vi "Instrument.TestLauncher.vi"(8 "error in (no error)":errorcluster, 10 "Debug Mode?":bool=TRUE) -> (0 "error out":errorcluster)   [LabVIEW 2019, in "Instrument.lvclass"]
uses:
  Instrument.lvclass
  <vilib>/JKI/JKI SMO/SMO/Typedefs/SMOState --Enum.ctl
  C:/Program Files (x86)/National Instruments/LabVIEW 2019/vi.lib/JKI/JKI SMO/SMO/SMO.lvclass
  <vilib>/JKI/JKI SMO/SMO/SMO.lvclass/SMO.ctl
  <vilib>/JKI/JKI SMO/SMO/Private/ReftoDVR--SMO.vi
  <vilib>/JKI/JKI SMO/SMO/SMO.lvclass
panel:
  out "SMO State":T1=enum."Stopped"
  in  "Stop":bool
  # "Instrument SMO Test Launcher"
  # "For instructions on how to use the JKI State Machine Objects, examples and video tutorials, visit:\nhttp://jki.net/state-machine-objects/\n\nJKI State Machine Objects™\nhttp://jki.net/state-machine-objects/\nCopyright (C) 2005-2015, JKI <info@jki.net>\nALL RIGHTS RESERVED"
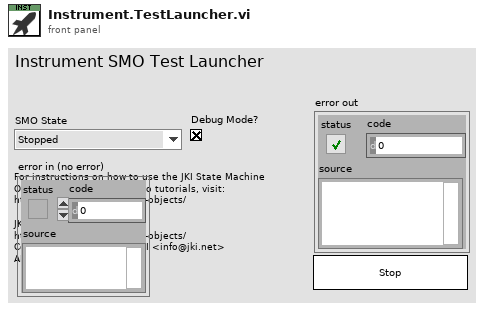
[diagram p1: front panel]
types:
  T1 = typedef "SMO.lvclass/SMOState --Enum.ctl" = enum16{"unknown", "Created", "Started", "Stopped"}
  T2 = typedef "SMO.lvclass/Public Events.ctl" = cluster{"Error":refnum<user-event>, "State":refnum<user-event>, "Reserve State":refnum<user-event>}
  T3 = cluster{"Event Registration Refnum":refnum<event-registration>}
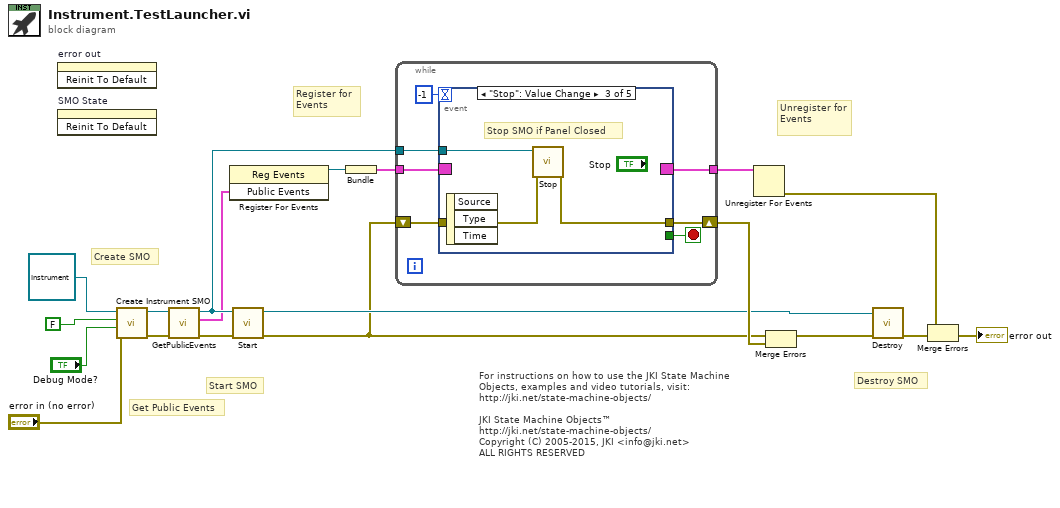
[diagram p0: block diagram]
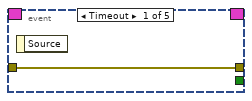
[diagram p2: hidden frame]
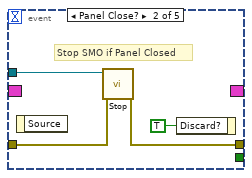
[diagram p3: hidden frame]
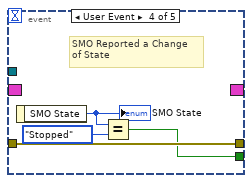
[diagram p4: hidden frame]
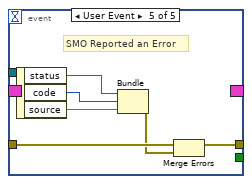
[diagram p5: hidden frame]
diagram:
  # "For instructions on how to use the JKI State Machine Objects, examples and video tutorials, visit:\nhttp://jki.net/state-machine-objects/\n\nJKI State Machine Objects™\nhttp://jki.net/state-machine-objects/\nCopyright (C) 2005-2015, JKI <info@jki.net>\nALL RIGHTS RESERVED"
  # "Get Public Events"
  # "Start SMO"
  # "Destroy SMO"
  # "Create SMO"
  # "Unregister for Events"
  # "Register for Events"
  n1 = invoke on="error out" class="Clust (strict)" method="Reinit To Default"() -> ()  [unwired: 3 in, 3 out]
  n2 = invoke on="SMO State" class="Enum (strict)" method="Reinit To Default"() -> ()  [unwired: 3 in, 3 out]
  n3 = call-dynamic "Create Instrument SMO.vi"("error in (no error)"="error in (no error)", "Debug Mode? [F]"="Debug Mode?", "Configuration Window? [T]"=FALSE ("Configuration Window?"), "Instrument in"=refnum<class "Instrument.lvclass"> refnum ("SMO.Template.lvclass")) -> ("error out"=w11:errorcluster, "Instrument out"=w12:refnum<class "Instrument.lvclass">)  [unwired: 6 in]
  n4 = call <vilib>:"GetPublicEvents.vi"("error in (no error)"=w11, "SMO"=w12) -> ("error out"=w10:errorcluster, "Public Events"=w8:T2, "SMO out"=w9:refnum<class "Instrument.lvclass">)  [unwired: 7 in]
  n5 = register-events(w8) -> (reference out=w7:refnum<event-registration>)  [unwired: 2 in, 1 out]
  n6 = call <vilib>:"Start.vi"("error in (no error)"=w10, "SMO"=w9) -> ("error out"=w2:errorcluster, "SMO out"=w5:refnum<class "Instrument.lvclass">)  [unwired: 8 in]
  n7 = Bundle("Event Registration Refnum"=w7) -> (w18:T3)  [unwired: 1 in]
  n8 = while {
    shift-right: [w25] -> w17
    shift-left: w2 -> [w24]
    tunnel: w18 -> [w23]
    tunnel: [w22] -> w19
    tunnel: w9 -> [w21]
    stop <- w26 stop-if-true
    n9 = event shown="[2] \"Stop\": Value Change" {
      selector: w23 -> [_ _ _ _ _]
      dyn-events: [_ _ _ _ _] -> w22
      timeout: -1 -> [_ _ _ _ _]
      tunnel: [_ _ _ w35 _] -> w26
      tunnel: w21 -> [_ w31 w34 _ _]
      tunnel: [w27 w30 w33 w38 w42] -> w25
      tunnel: w24 -> [w27 w29 w32 w38 w40]
      event Timeout {
        n10 = event-data() -> ()  [unwired: 1 in, 1 out]
      }
      event Panel Close? {
        # "Stop SMO if Panel Closed"
        n11 = event-data() -> ()  [unwired: 1 in, 1 out]
        n12 = call <vilib>:"Stop.vi"("error in (no error)"=w29, "SMO"=w31) -> ("error out"=w30:errorcluster)  [unwired: 8 in, 1 out]
        n13 = event-data("Discard?"=TRUE ("OK")) -> ()  [unwired: 1 in, 1 out]
      }
      event "Stop": Value Change {
        # "Stop SMO if Panel Closed"
        n14 = event-data() -> ()  [unwired: 1 in, 3 out]
        n15 = call <vilib>:"Stop.vi"("error in (no error)"=w32, "SMO"=w34) -> ("error out"=w33:errorcluster)  [unwired: 8 in, 1 out]
      }
      event User Event {
        # "SMO Reported a Change\nof State"
        n16 = event-data() -> ("SMO State"=w37:T1)  [unwired: 1 in]
        "SMO State" <- w37
        n17 = Equal?(x=w37, y=SMOState_--Enum."Stopped") -> (x = y?=w35:bool)
      }
      event User Event {
        # "SMO Reported an Error"
        n18 = event-data() -> ("status"=w41:bool, "code"=w44:i32, "source"=w43:string)  [unwired: 1 in]
        n19 = Bundle("status"=w41, "code"=w44, "source"=w43) -> (w39:errorcluster)  [unwired: 1 in]
        n20 = Merge Errors(w40, w39) -> (w42:errorcluster)
      }
    }
  }
  n21 = Unregister For Events(event registration refnum=w19) -> (error out=w16:errorcluster)  [unwired: 1 in]
  n22 = Merge Errors(w2, w17) -> (w13:errorcluster)
  n23 = call <vilib>:"Destroy.vi"("error in (no error)"=w13, "SMO"=w5) -> ("error out"=w14:errorcluster)  [unwired: 9 in]
  n24 = Merge Errors(w16, w14) -> (→"error out":errorcluster)
